vi "ISEG_HVChannel.get data to modify.vi"(0 "i ref in":refnum<vi>, 3 "ms timeout (10000)":i32=10000, 5 "error in (no error)":errorcluster) -> (14 "i ref out":refnum<vi>, 16 "i attribute":T1 {"Channel Array"."EventMask"."EventMask" format="%.0b"; "Channel Array"."Status"."Status" format="%.0b"}, 17 "timed out":bool, 19 "error out":errorcluster)   [LabVIEW 2014, in "ISEG_HVChannel.lvlib"]
doc: "Reads the attribute data of the object after the access to the data has been locked by the \"acquire\" method. If the attribute data has been locked already, this methods waits until the attribute data is unlocked or there is a timeout.\n\nThe attribute data must be unlocked using the methods \"release\" or \"set modified data\".\n\nLicense Agreement for this software:\n\nCopyright (C)\nGesellschaft für Schwerionenforschung, GSI\nPlanckstr. 1\n64291 Darmstadt\nGermany\n\nContact: D.Beck@gsi.de \n\nThis program is free software; you can redistribute it and/or modify it under the terms of the GNU General Public License as published by the Free Software Foundation; either version 2 of the license, or (at your option) any later version.\n\nThis program is distributed in the hope that it will be useful, but WITHOUT ANY WARRANTY; without even the implied warranty of MERCHANTABILITY or FITNESS FOR A PARTICULAR PURPOSE. See the GNU General License for more details (http://www.gnu.org).\n\nGesellschaft für Schwerionenforschung, GSI\nPlanckstr. 1, 64291 Darmstadt, Germany\nFor all questions and ideas contact: M.Richter@gsi.de, H.Brand@gsi.de or D.Beck@gsi.de.\nLast update: 17-JUN-2004"
uses:
  ISEG_HVChannel.lvlib
  ISEG_HVChannel.i attribute.ctl
  ISEG_HVChannel.DIM Status.ctl
  CS_Core/CSObj/CSObj.lvlib
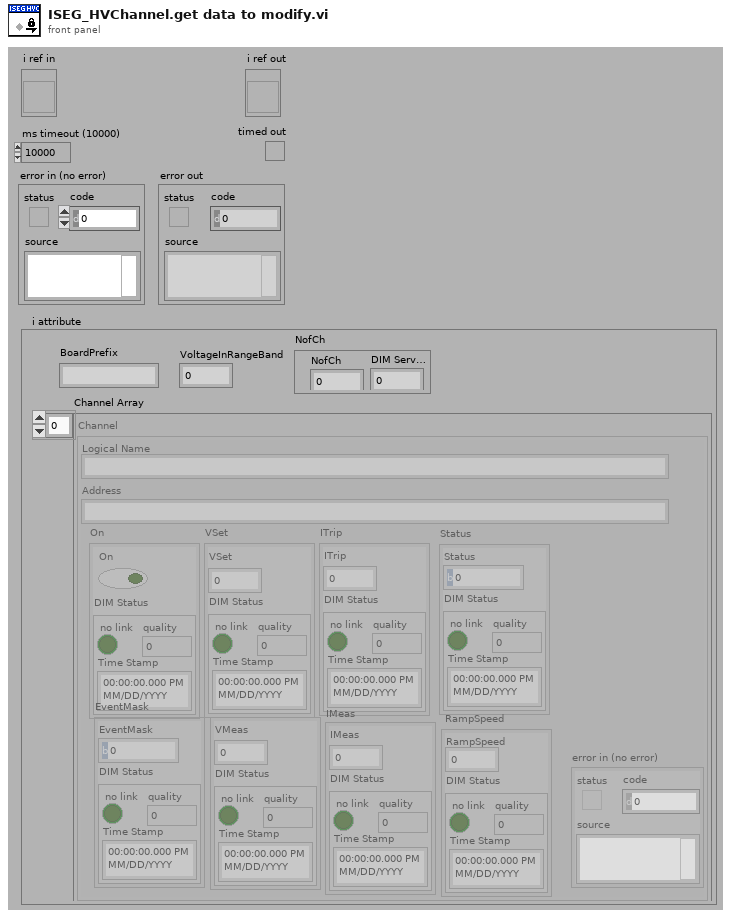
[diagram p1: front panel]
types:
  T1 = typedef "ISEG_HVChannel.lvlib/ISEG_HVChannel.i attribute.ctl" = cluster{"Channel Array":cluster{"Logical Name":string, "Address":string, "error in (no error)":errorcluster, "Status":cluster{"Status":i16, "DIM Status":T2}, "On":cluster{"On":bool, "DIM Status":T2}, "VMeas ":cluster{"VMeas":dbl, "DIM Status":T2}, "VSet ":cluster{"VSet":dbl, "DIM Status":T2}, "ITrip ":cluster{"ITrip":dbl, "DIM Status":T2}, "IMeas":cluster{"IMeas":dbl, "DIM Status":T2}, " RampSpeed":cluster{"RampSpeed":dbl, "DIM Status":T2}, "EventMask ":cluster{"EventMask":i16, "DIM Status":T2}}[], "VoltageInRangeBand":dbl, "NofCh":cluster{"NofCh":i32, "DIM Service":i32}, "BoardPrefix":string}
  T2 = typedef "ISEG_HVChannel.lvlib/ISEG_HVChannel.DIM Status.ctl" = cluster{"no link":bool, "quality":i32, "Time Stamp":timestamp}
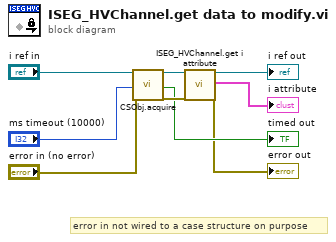
[diagram p0: block diagram]
diagram:
  # "error in not wired to a case structure on purpose"
  n1 = call "CSObj.acquire.vi"("i ref in"="i ref in", "ms timeout (10000)"="ms timeout (10000)", "error in (no error)"="error in (no error)") -> ("i ref out"=w8:refnum<vi>, "timed out"=→"timed out":bool, "error out"=w5:errorcluster)  [unwired: 14 in]
  n2 = call "ISEG_HVChannel.get i attribute.vi"("i ref in"=w8, "error in (no error)"=w5) -> ("i ref out"=→"i ref out":refnum<vi>, "i attribute"=→"i attribute":T1, "error out"=→"error out":errorcluster)  [unwired: 15 in]
